vi "Read Until Timeout.vi"(8 "error in (no error)":errorcluster, 11 "FTP in":refnum<class "FTP.lvclass">) -> (0 "error out":errorcluster, 3 "FTP out":refnum<class "FTP.lvclass">)   [LabVIEW 2017, in "FTP_UpgradeCSMF.lvlib" / "FTP.lvclass"]
uses:
  FTP.lvclass
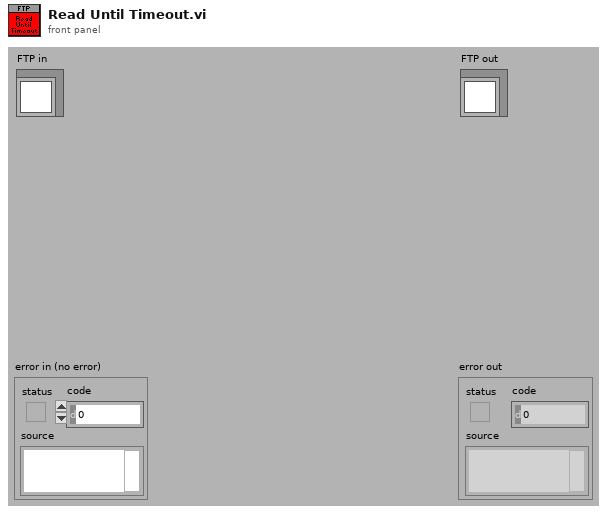
[diagram p1: front panel]
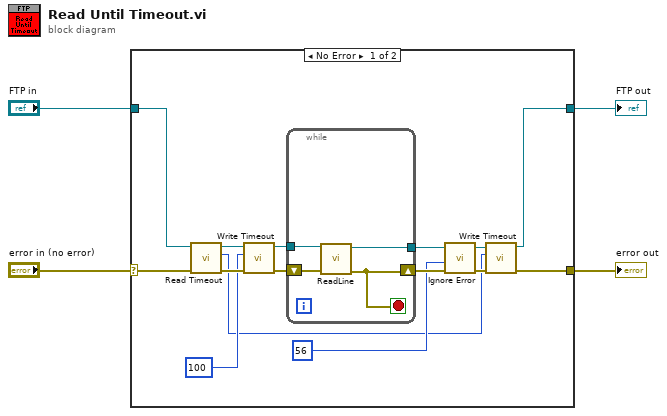
[diagram p0: block diagram]
diagram:
  n1 = case shown="No Error" "error in (no error)" {
    selector: "error in (no error)" -> [w6 w24]
    tunnel: [w5 w24] -> w3
    tunnel: [w7 w23] -> w1
    tunnel: "FTP in" -> [w8 w23]
    frame No Error {
      n2 = call "Read Timeout.vi"("error in (no error)"=w6, "FTP in"=w8) -> ("error out"=w15:errorcluster, "Timeout"=w9:i32, "FTP out"=w16:refnum<class "FTP.lvclass">)  [unwired: 7 in]
      n3 = call "Write Timeout.vi"("error in (no error)"=w15, "Timeout"=100, "FTP in"=w16) -> ("error out"=w13:errorcluster, "FTP out"=w14:refnum<class "FTP.lvclass">)  [unwired: 7 in]
      n4 = while {
        tunnel: w14 -> [w21]
        tunnel: [w20] -> w11
        shift-right: [w19] -> w18
        shift-left: w13 -> [w22]
        stop <- w19 stop-if-true
        n5 = call "ReadLine.vi"("error in (no error)"=w22, "FTP in"=w21) -> ("error out"=w19:errorcluster, "FTP out"=w20:refnum<class "FTP.lvclass">)  [unwired: 5 in, 3 out]
      }
      n6 = call "Ignore Error.vi"("error in"=w18, "code"=56) -> ("error out"=w12:errorcluster)  [unwired: 9 in]
      n7 = call "Write Timeout.vi"("error in (no error)"=w12, "Timeout"=w9, "FTP in"=w11) -> ("error out"=w5:errorcluster, "FTP out"=w7:refnum<class "FTP.lvclass">)  [unwired: 7 in]
    }
    frame Error {
    }
  }
  "error out" <- w3
  "FTP out" <- w1
